vi "Measurement Logic.vi"(8 "error in":errorcluster, 9 "measurement configuration":T2={"Resource Name"="", "Measure Trigger Source"="", "Run Until"=inf, "Current Limit"=32.0, "Voltage Level"=64.0, "Current Limit Range"=0.1, "Voltage Level Range"=5.0, "Aperture Time"=1.2, "Current Unit"="Lorem ipsum dolor sit", "Delimited Text"=","} {"Aperture Time" min=1.0 step=1.0 format="%#_g Samples"; "Voltage Level Range" format="%#_6pV"; "Current Limit Range" format="%#_6pA"; "Voltage Level" format="%#_6pV"; "Run Until" format="%#_6ps"}, 10 "measure call context in":refnum<class "Measure Call Context.lvclass">) -> (0 "error out":errorcluster, 1 "measurement results":T1={"Text Result"="Empty", "Measured Voltages"=[0.0], "Measured Currents"=[0.0], "Actual Aperture Time"=0.0, "In Compliance"=[], "Any In Compliance?"=FALSE} {"Actual Aperture Time" format="%#_6ps"}, 2 "measure call context out":refnum<class "Measure Call Context.lvclass">)   [LabVIEW 2025, in "DCPower Single Meas Per Trigger.lvclass"]
doc: "Contains the core logic for executing the measurement."
uses:
  DCPower Single Meas Per Trigger.lvclass
  DCPower Single Meas Per Trigger.lvclass/DCPower Single Meas Per Trigger.ctl
  <vilib>/Plug-In SDKs/Measurements/Measure Call Context/Measure Call Context.lvclass
  <vilib>/Plug-In SDKs/Sessions/niDCPower/NI Session Management niDCPower.lvlib
  <vilib>/Plug-In SDKs/Clients/Session Management V1/Session Reservation/Session Reservation.lvclass
  <vilib>/Plug-In SDKs/Sessions/niDCPower/Initialize Sessions - 1Sess.vi
  <vilib>/Plug-In SDKs/Measurements/Measure Call Context/Reserve Sessions - 1Pin.vi
  Measurement Configuration.ctl
  Measurement Results.ctl
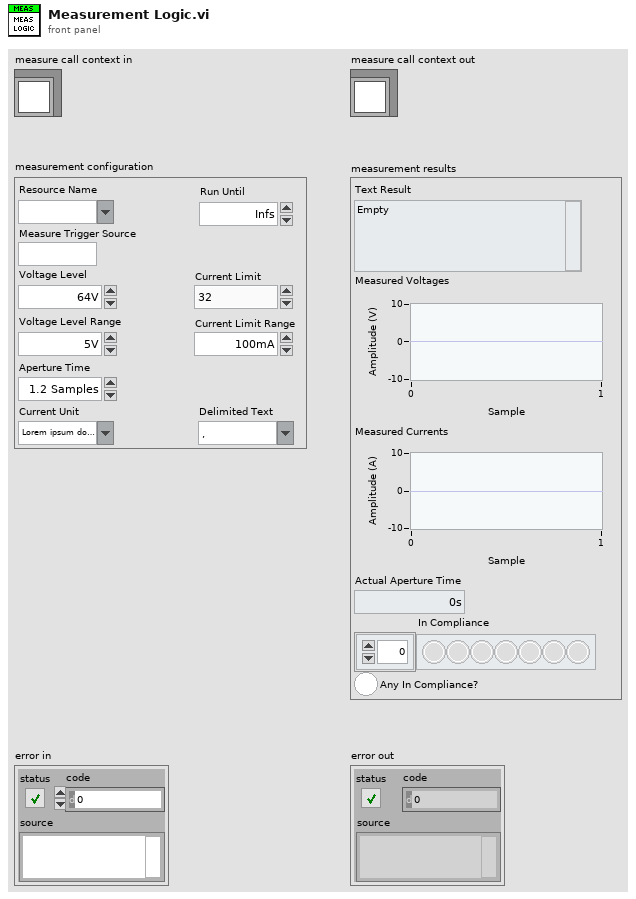
[diagram p1: front panel]
types:
  T1 = typedef "DCPower Single Meas Per Trigger.lvclass/Measurement Results.ctl" = cluster{"Text Result":string, "Measured Voltages":dbl[], "Measured Currents":dbl[], "Actual Aperture Time":dbl, "In Compliance":bool[], "Any In Compliance?":bool}
  T2 = typedef "DCPower Single Meas Per Trigger.lvclass/Measurement Configuration.ctl" = cluster{"Resource Name":string, "Measure Trigger Source":string, "Run Until":dbl, "Current Limit":dbl, "Voltage Level":dbl, "Current Limit Range":dbl, "Voltage Level Range":dbl, "Aperture Time":dbl, "Current Unit":string, "Delimited Text":string}
  T3 = typedef "Event Messenger-bool.lvlib/))Channel.ctl" = refnum<queue>
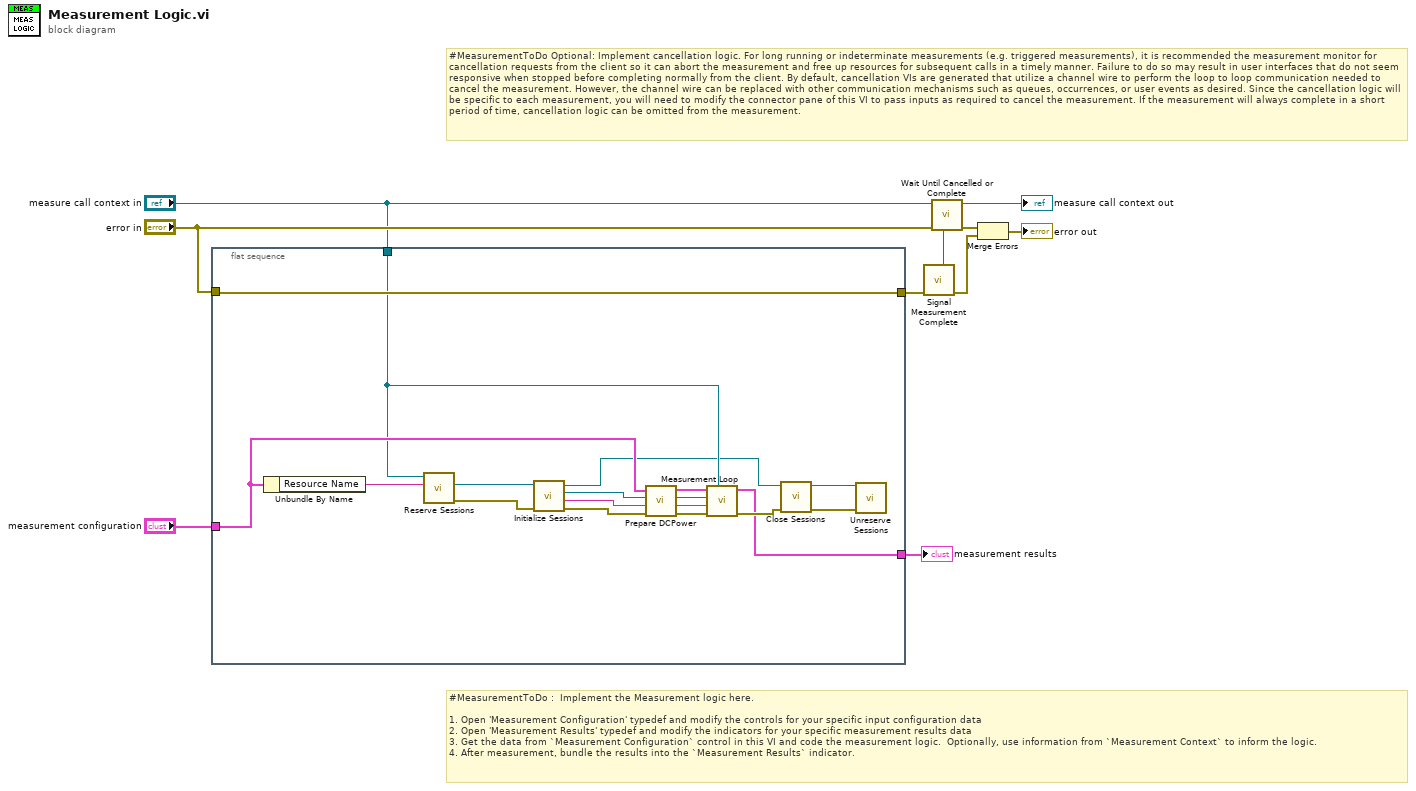
[diagram p0: block diagram]
diagram:
  # "#MeasurementToDo Optional: Implement cancellation logic. For long running or indeterminate measurements (e.g. triggered measurements), it is recommended the measurement monitor for cancellation requests from the client so it can abort the measurement and free up resources for subsequent calls in a timely manner. Failure to do so may result in user interfaces that do not seem responsive when stopped before completing normally from the client. By default, cancellation VIs are generated that utilize a channel wire to perform the loop to loop communication needed to cancel the measurement. However, the channel wire can be replaced with other communication mechanisms such as queues, occurrences, or user events as desired. Since the cancellation logic will be specific to each measurement, you will need to modify the connector pane of this VI to pass inputs as required to cancel the measurement. If the measurement will always complete in a short period of time, cancellation logic can be omitted from the measurement."
  # "#MeasurementToDo :  Implement the Measurement logic here.\n\n1. Open 'Measurement Configuration' typedef and modify the controls for your specific input configuration data\n2. Open 'Measurement Results' typedef and modify the indicators for your specific measurement results data\n3. Get the data from `Measurement Configuration` control in this VI and code the measurement logic.  Optionally, use information from `Measurement Context` to inform the logic.\n4. After measurement, bundle the results into the `Measurement Results` indicator."
  n1 = flat-sequence {
    tunnel: "measurement configuration" -> [w18]
    tunnel: "error in" -> [w28]
    tunnel: [w28] -> w7
    tunnel: "measure call context in" -> [w14]
    tunnel: [w13] -> w1
    frame #0 {
      n2 = Unbundle By Name(w18) -> ("Resource Name"=w27:string)
      n3 = call-poly <vilib>:"Reserve Sessions.vi"("pin or relay name"=w27, "measurement context in"=w14) -> ("error out"=w11:errorcluster, "session reservation out"=w26:refnum<class "Session Reservation.lvclass">)  [unwired: 7 in, 1 out]
      n4 = call-poly <vilib>:"Initialize Sessions.vi"("error in"=w11, "session reservation in"=w26) -> ("error out"=w22:errorcluster, "channel list"=w20:string, "session"=w21:refnum<k15>, "session reservation out"=w12:refnum<class "Session Reservation.lvclass">)  [unwired: 6 in]
      n5 = call "Prepare DCPower.vi"("error in"=w22, "Channel List in"=w20, "Instrument Handle in"=w21, "Measurement Configuration in"=w18) -> ("error out"=w23:errorcluster, "Channel List out"=w15:string, "Instrument Handle out"=w17:refnum<k15>, "Measurement Configuration out"=w16:T2)  [unwired: 4 in]
      n6 = call "Measurement Loop.vi"("measure call context in"=w14, "error in"=w23, "channel list"=w15, "instrument handle"=w17, "Measurement Configuration"=w16) -> ("error out"=w19:errorcluster, "Measurement Results"=w13:T1)  [unwired: 5 in]
      n7 = call <vilib>:"Close Sessions.vi"("error in"=w19, "session reservation in"=w12) -> ("error out"=w25:errorcluster, "session reservation out"=w24:refnum<class "Session Reservation.lvclass">)  [unwired: 8 in]
      n8 = call <vilib>:"Unreserve Sessions.vi"("error in"=w25, "session reservation in"=w24) -> ()  [unwired: 9 in, 1 out]
    }
  }
  n9 = call "Signal Measurement Complete.vi"("error in (no error)"=w7) -> ("error out"=w5:errorcluster, "done channel"=w6:T3)  [unwired: 9 in]
  n10 = call "Wait Until Cancelled or Complete.vi"("done channel"=w6, "error in (no error)"="error in", "measure call context in"="measure call context in") -> ("error out"=w4:errorcluster, "measure call context out"=→"measure call context out":refnum<class "Measure Call Context.lvclass">)  [unwired: 7 in]
  n11 = Merge Errors(w4, w5) -> (→"error out":errorcluster)
  "measurement results" <- w1
